vi "RawSimultaneousRead.vi"() -> ()   [LabVIEW 2017]
uses:
  <vilib>/rvi/Emulation/niFpgaGetClockAttributes.vi
  <vilib>/rvi/Emulation/niFpgaSctlEmulationGetInTimedLoop.vi
  <vilib>/rvi/Emulation/niFpgaEmulationReportErrorSimple.vi
  <vilib>/rvi/eio/common/nirviEmuTemplateMethod_errors.vi
  <vilib>/rvi/Emulation/niFpgaCriticalErrorInLSC.vi
  <vilib>/eio/EIONode/EIONode.xnode
panel:
  out "RawValues":i16[](array[numeric])
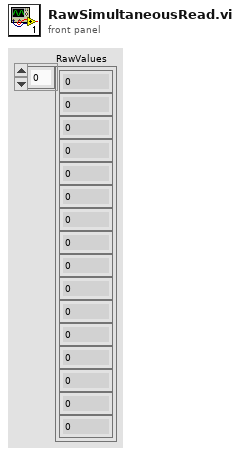
[diagram p1: front panel]
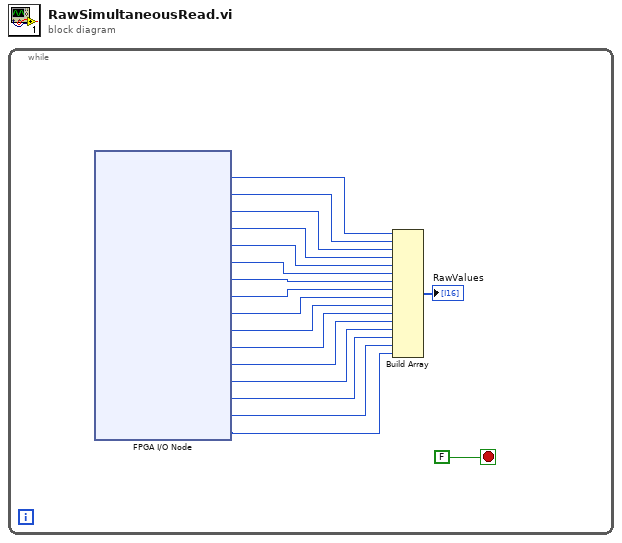
[diagram p0: block diagram]
diagram:
  n1 = while {
    stop <- FALSE ("stop") stop-if-true
    n2 = xnode "FPGA I/O Node"() -> ("I0_BuckBoost"=w18:i16, "I1_BuckBoost"=w17:i16, "I2_BuckBoost"=w16:i16, "Vgrid_BuckBoost"=w15:i16, "VDCLink_BuckBoost"=w14:i16, "V0_BuckBoost"=w13:i16, "V1_BuckBoost"=w12:i16, "V2_BuckBoost"=w11:i16, "Iu_AFE"=w10:i16, "Iv_AFE"=w9:i16, "Iw_AFE"=w8:i16, "VLoad_BuckBoost"=w7:i16, "Vu_AFE"=w6:i16, "Vv_AFE"=w5:i16, "Vw_AFE"=w4:i16, "VDCLink_AFE"=w3:i16)  [unwired: 16 in, 16 out]
    n3 = Build Array(w18, w17, w16, w15, w14, w13, w12, w11, w10, w9, w8, w7, w6, w5, w4, w3) -> (→"RawValues":i16[])
  }
